vi "Functional Global Variable.vi"(9 "Action":T1, 11 "Mode":cluster{"Run":bool, "Hold":bool, "Off":bool}={"Run"=FALSE, "Hold"=FALSE, "Off"=TRUE}) -> (3 "Mode":cluster{"Run":bool, "Hold":bool, "Off":bool}={"Run"=FALSE, "Hold"=FALSE, "Off"=TRUE})   [LabVIEW 2012]
uses:
  Action Items.ctl
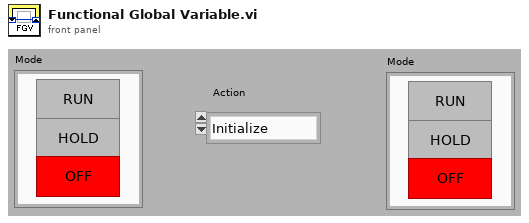
[diagram p1: front panel]
types:
  T1 = typedef "Action Items.ctl" = enum16{"Initialize", "Get", "Increment"}
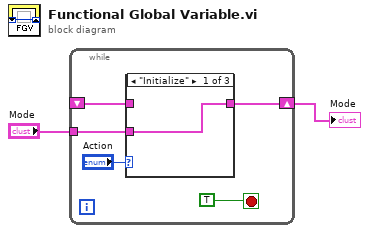
[diagram p0: block diagram]
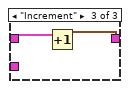
[diagram p3: hidden frame]
diagram:
  n1 = while {
    shift-right: [w7] -> w1
    shift-left: _ -> [w6]
    tunnel: "Mode" -> [w3]
    stop <- TRUE ("stop") stop-if-true
    n2 = case shown="\"Initialize\"" "Action" {
      tunnel: [w8 w9 w10] -> w7
      tunnel: w6 -> [_ w9 w11]
      tunnel: w3 -> [w8 _ _]
      frame "Initialize" {
      }
      frame "Get" {
      }
      frame "Increment" {
        n3 = Increment(x=w11) -> (x+1=w10:cluster{"Run":dbl, "Hold":dbl, "Off":dbl})
      }
    }
  }
  "Mode" <- w1
